vi "Init Client.vi"(7 "Client TLS Config (Disabled)":T1, 8 "error in (no error)":errorcluster, 10 "Port":u16, 11 "Host":string) -> (0 "error out":errorcluster, 3 "TCP Comm":T3)   [LabVIEW 2020, in "TCP Comms.lvlib"]
doc: "Initializes a TCP Client that will connect to the specified server once <b>Open.vi</b> is called. Once Open is called, the client will continually attempt to connect to the server and if connection is lost it will reconnect. The status of the connection can be checked with <b>Get State.vi</b> Once the connection is no longer needed, call <b>Close.vi</b> to close the client connection. To cleanup the client and release all resources call <b>Stop.vi</b>"
uses:
  TCP Comms.lvlib
  TCP Comm.ctl
  Ref Data.ctl
  State.ctl
  Client TLS Config.ctl
  Cert Chain.ctl
  TLS Config.ctl
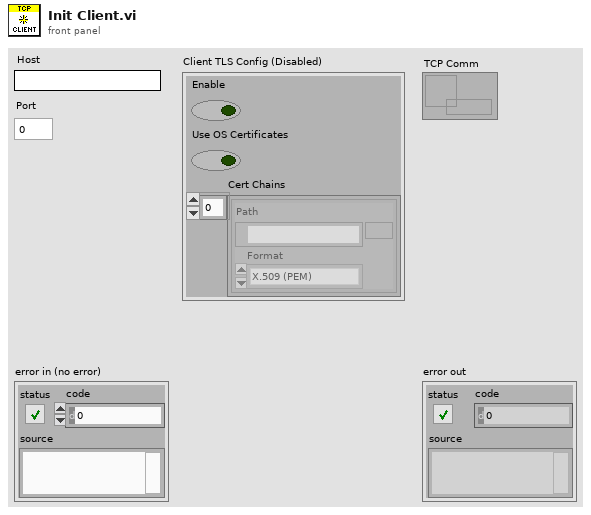
[diagram p1: front panel]
types:
  T1 = typedef "TCP Comms.lvlib/Client TLS Config.ctl" = cluster{"Enable":bool, "Use OS Certificates":bool, "Cert Chains":T2[]}
  T2 = typedef "TCP Comms.lvlib/Cert Chain.ctl" = cluster{"Path":path, "Format":enum32{"X.509 (PEM)"}}
  T3 = typedef "TCP Comms.lvlib/TCP Comm.ctl" = refnum<data-value>
  T4 = typedef "TCP Comms.lvlib/TLS Config.ctl" = cluster{"TLS Enabled":bool, "Use OS Cert Chains":bool, "Private Key Path":path, "Private Key Format":enum32{"PKCS#8 (PEM)", "PKCS#8 (DER)"}, "Private Key Password":string, "Private Key Cert Chain":T2, "Cert Chains":T2[]}
  T5 = typedef "TCP Comms.lvlib/Ref Data.ctl" = cluster{"TCP":refnum<k5>, "State":T6, "Server":bool, "Host":string, "Port":u16, "Listener":refnum<k5>, "Start":bool, "Disconnect":bool, "TCP Valid":bool, "TLS Enabled":bool, "Immutable TLS":refnum<k36>, "Certificate DN":string}
  T6 = typedef "TCP Comms.lvlib/State.ctl" = enum16{"Idle", "Starting", "Connecting", "Connected", "Disconnecting", "Stopped"}
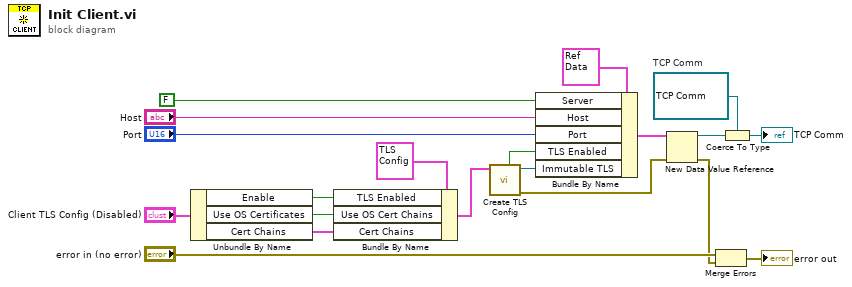
[diagram p0: block diagram]
diagram:
  w11 = T3 refnum  # TCP Comm
  n1 = Unbundle By Name("Client TLS Config (Disabled)") -> ("Enable"=w3:bool, "Use OS Certificates"=w2:bool, "Cert Chains"=w1:T2[])
  n2 = Bundle By Name(cluster=T4 {"TLS Enabled"=FALSE, "Use OS Cert Chains"=FALSE, "Private Key Path"=path "", "Private Key Format"=enum."PKCS#8 (PEM)", "Private Key Password"="", "Private Key Cert Chain"={"Path"=path "", "Format"=enum."X.509 (PEM)"}, "Cert Chains"=[]} ("TLS Config"), "TLS Enabled"=w3, "Use OS Cert Chains"=w2, "Cert Chains"=w1) -> (w4:T4)
  n3 = call "Create TLS Config.vi"("TLS Config"=w4) -> ("error out"=w7:errorcluster, "Immutable TLS"=w9:refnum<k36>, "TLS Enabled"=w8:bool)  [unwired: 8 in]
  n4 = Bundle By Name(cluster=T5 {"TCP"=refnum, "State"=enum."Idle", "Server"=FALSE, "Host"="", "Port"=0, "Listener"=refnum, "Start"=FALSE, "Disconnect"=FALSE, "TCP Valid"=FALSE, "TLS Enabled"=FALSE, "Immutable TLS"=refnum, "Certificate DN"=""} ("Ref Data"), "Server"=FALSE, "Host"="Host", "Port"="Port", "TLS Enabled"=w8, "Immutable TLS"=w9) -> (w17:T5)
  n5 = New Data Value Reference(data value=w17, error in=w7) -> (data value reference=w13:refnum<data-value>, error out=w15:errorcluster)
  n6 = Merge Errors("error in (no error)", w15) -> (→"error out":errorcluster)
  n7 = Coerce To Type(0:w13, 1:w11) -> (2:→"TCP Comm":T3)
